vi "FindComponentActorCluster.vi"(10 "Alias":string, 11 "Actor":refnum<class "Actor.lvclass">) -> (2 "ComponentActorCluster":T1, 3 "Found":bool)   [LabVIEW 2020, in "jettl.lvlib"]
uses:
  jettl.lvlib
  Actor/Actor.lvclass
  Message/Message.lvclass
  MessageSet.ctl
  MessagesCluster.ctl
  MessageCluster.ctl
  ActorCluster.ctl
  ActorTypeEnum.ctl
  TellComponentMessageSetMap.ctl
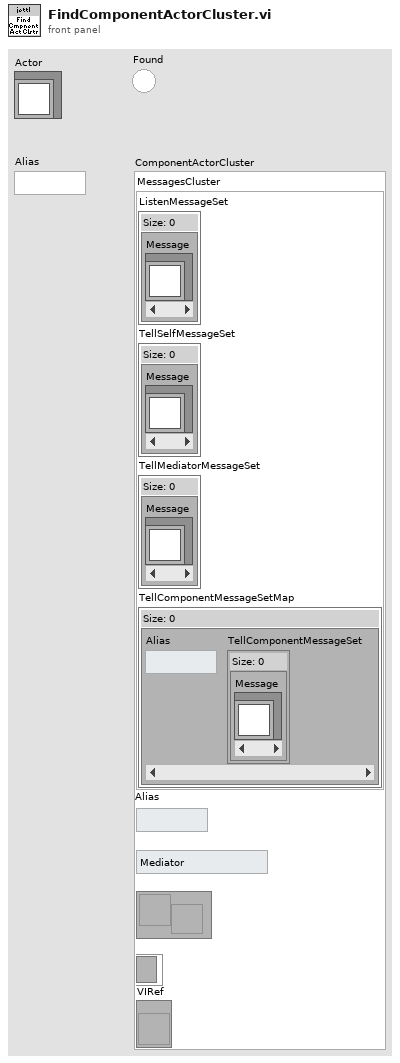
[diagram p1: front panel]
types:
  T1 = typedef "jettl.lvlib/ActorCluster.ctl" = cluster{"MessagesCluster":T2, "Alias":string, "ActorTypeEnum":T5, "MessageClusterDVREvent":refnum<user-event>, "EventRegistrationRef":refnum<event-registration>, "VIRef":refnum<vi>}
  T2 = typedef "jettl.lvlib/MessagesCluster.ctl" = cluster{"ListenMessageSet":T3, "TellSelfMessageSet":T3, "TellMediatorMessageSet":T3, "TellComponentMessageSetMap":T4}
  T3 = typedef "jettl.lvlib/MessageSet.ctl" = set{refnum<class "Message.lvclass">}
  T4 = typedef "jettl.lvlib/TellComponentMessageSetMap.ctl" = map{string, T3}
  T5 = typedef "jettl.lvlib/ActorTypeEnum.ctl" = enum16{"Mediator", "Component"}
  T6 = typedef "jettl.lvlib/BaseCluster.ctl" = cluster{"LifecycleEnum":T7, "MainCluster":T8, "SelfActorCluster":T1, "MediatorActorCluster":T1, "ComponentActorClusterMap":T9}
  T7 = typedef "jettl.lvlib/LifecycleEnum.ctl" = enum16{"Initializing", "SettingUp", "Starting", "Running", "Stopping", "TearingDown", "Terminated"}
  T8 = typedef "jettl.lvlib/MainCluster.ctl" = cluster{"PreSetupClusterQueue":refnum<queue>, "BeginSetupQueue":refnum<queue>, "SetupErrorQueue":refnum<queue>, "BeginStartQueue":refnum<queue>}
  T9 = typedef "jettl.lvlib/ComponentActorClusterMap.ctl" = map{string, T1}
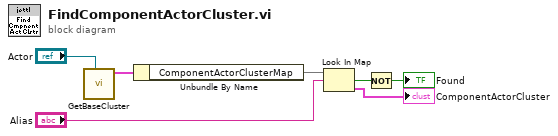
[diagram p0: block diagram]
diagram:
  n1 = call-dynamic "GetBaseCluster.vi"("Actor"="Actor") -> ("BaseCluster"=w3:T6)  [unwired: 10 in]
  n2 = Unbundle By Name(w3) -> ("ComponentActorClusterMap"=w1:T9)
  n3 = Look In Map(map=w1, key="Alias") -> (key not found?=w5:bool, value=→"ComponentActorCluster":T1)  [unwired: 1 in]
  n4 = Not(x=w5) -> (.not. x?=→"Found":bool)
